vi "Read Encoders.vi"(8 "Reset":bool, 10 "Right Encoder":T2, 11 "Left Encoder":T2) -> (0 "Encoder Values":T1, 2 "Right Encoder Out":T2, 3 "Left Encoder Out":T2)   [LabVIEW 2013]
uses:
  <vilib>/Rock Robotics/WPI/Encoder/WPI_EncoderDevRef.ctl
  <vilib>/Rock Robotics/SystemInterfaces/Encoder/FPGA_EncoderIdx.ctl
  <vilib>/Rock Robotics/SystemInterfaces/Counter/FPGA_CounterCtrSystemIndex.ctl
  <vilib>/Rock Robotics/WPI/Encoder/WPI_EncoderType.ctl
  Encoder Values.ctl
  <vilib>/addons/control/pid/pid.llb/PID Control Input Filter (DBL).vi
  <vilib>/addons/control/pid/NI_PID_pid.lvlib
panel:
  in  "Left constant":dbl=0.00724
  in  "Right constant":dbl=0.00724
  in  "Right tick constant":dbl=0.697
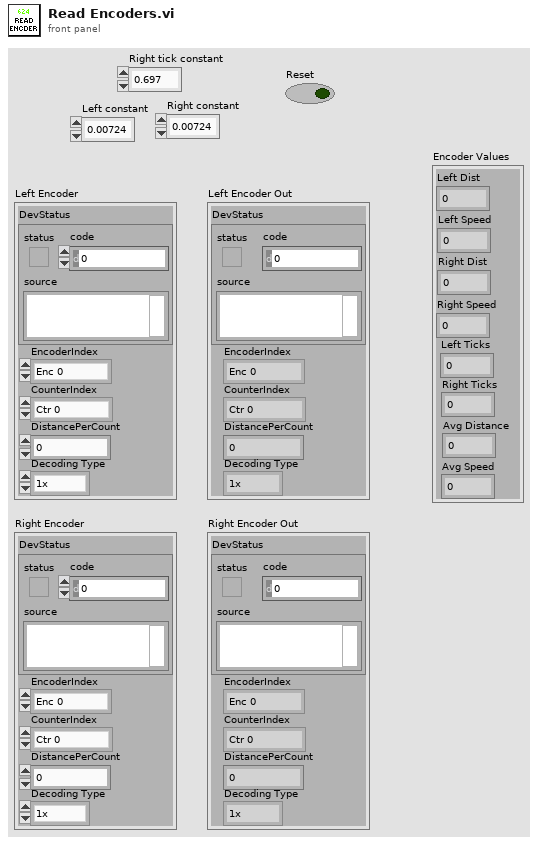
[diagram p1: front panel]
types:
  T1 = typedef "Encoder Values.ctl" = cluster{"Left Dist":dbl, "Left Speed":dbl, "Right Dist":dbl, "Right Speed":dbl, "Left Ticks":dbl, "Right Ticks":dbl, "Avg Distance":dbl, "Avg Speed":dbl}
  T2 = typedef "WPI_EncoderDevRef.ctl" = cluster{"DevStatus":errorcluster, "EncoderIndex":T3, "CounterIndex":T4, "DistancePerCount":dbl, "Decoding Type":T5}
  T3 = typedef "FPGA_EncoderIdx.ctl" = enum8{"Enc 0", "Enc 1", "Enc 2", "Enc 3", "Invalid"}
  T4 = typedef "FPGA_CounterCtrSystemIndex.ctl" = enum8{"Ctr 0", "Ctr 1", "Ctr 2", "Ctr 3", "Ctr 4", "Ctr 5", "Ctr 6", "Ctr 7", "Invalid"}
  T5 = typedef "WPI_EncoderType.ctl" = enum16{"1x", "2x", "4x"}
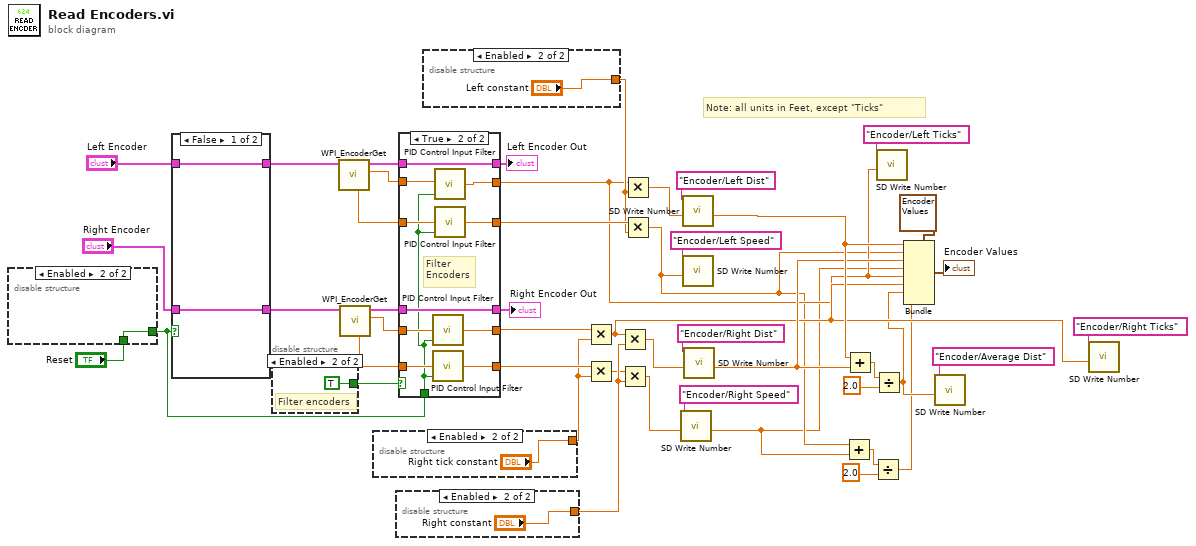
[diagram p0: block diagram]
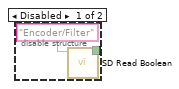
[diagram p2: hidden frame]
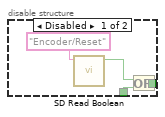
[diagram p3: hidden frame]
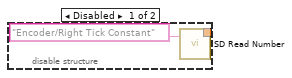
[diagram p4: hidden frame]
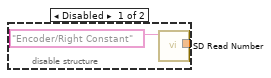
[diagram p5: hidden frame]
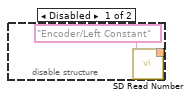
[diagram p6: hidden frame]
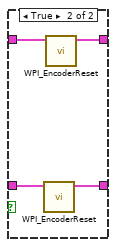
[diagram p7: hidden frame]
diagram:
  # "Note: all units in Feet, except \"Ticks\""
  n1 = disable-structure shown="Enabled" {
    disable-tunnel: "Reset" -> [w46 w48]
    disable-tunnel: [w44 w48] -> w7
    frame Disabled {
      n2 = call <vilib>:"SD Read Boolean.vi"("Name"="Encoder/Reset") -> ("Boolean"=w45:bool)  [unwired: 8 in, 2 out]
      n3 = Or(x=w45, y=w46) -> (x .or. y?=w44:bool)
    }
    frame Enabled {
    }
  }
  n4 = case shown="False" w7 {
    tunnel: [w49 w54] -> w8
    tunnel: [w50 w53] -> w9
    tunnel: "Left Encoder" -> [w50 w52]
    tunnel: "Right Encoder" -> [w49 w51]
    frame False {
    }
    frame True {
      n5 = call <vilib>:"WPI_EncoderReset.vi"("EncoderDevRef"=w51) -> ("EncoderDevRef"=w54:T2)  [unwired: 9 in, 1 out]
      n6 = call <vilib>:"WPI_EncoderReset.vi"("EncoderDevRef"=w52) -> ("EncoderDevRef"=w53:T2)  [unwired: 9 in, 1 out]
    }
  }
  n7 = disable-structure shown="Enabled" {
    disable-tunnel: [w55 TRUE ("Boolean")] -> w12
    frame Disabled {
      n8 = call <vilib>:"SD Read Boolean.vi"("Name"="Encoder/Filter") -> ("Boolean"=w55:bool)  [unwired: 8 in, 2 out]
    }
    frame Enabled {
      # "Filter encoders"
    }
  }
  n9 = call <vilib>:"WPI_EncoderGet.vi"("EncoderDevRef"=w9) -> ("Distance"=w33:dbl, "EncoderDevRef"=w36:T2, "Rate"=w34:dbl)  [unwired: 5 in, 3 out]
  n10 = call <vilib>:"WPI_EncoderGet.vi"("EncoderDevRef"=w8) -> ("Distance"=w32:dbl, "EncoderDevRef"=w35:T2, "Rate"=w31:dbl)  [unwired: 5 in, 3 out]
  n11 = disable-structure shown="Enabled" {
    disable-tunnel: [w58 "Right tick constant"] -> w24
    frame Disabled {
      n12 = call <vilib>:"SD Read Number.vi"("Name"="Encoder/Right Tick Constant") -> ("Numeric"=w58:dbl)  [unwired: 8 in, 2 out]
    }
    frame Enabled {
    }
  }
  n13 = disable-structure shown="Enabled" {
    disable-tunnel: [w61 "Right constant"] -> w27
    frame Disabled {
      n14 = call <vilib>:"SD Read Number.vi"("Name"="Encoder/Right Constant") -> ("Numeric"=w61:dbl)  [unwired: 8 in, 2 out]
    }
    frame Enabled {
    }
  }
  n15 = case shown="True" w12 {
    tunnel: w36 -> [w69 w80]
    tunnel: w35 -> [w66 w79]
    tunnel: [w69 w80] -> w15
    tunnel: [w66 w79] -> w16
    tunnel: w33 -> [w68 w78]
    tunnel: w34 -> [w67 w77]
    tunnel: [w67 w76] -> w30
    tunnel: [w68 w75] -> w19
    tunnel: w31 -> [w64 w74]
    tunnel: w32 -> [w65 w73]
    tunnel: [w65 w72] -> w23
    tunnel: [w64 w71] -> w26
    tunnel: w7 -> [_ w70]
    frame False {
      # "No filtering"
    }
    frame True {
      # "Filter\nEncoders"
      n16 = call-poly <vilib>:"PID Control Input Filter.vi"("reinitialize? (F)"=w70, "input"=w73) -> ("output"=w72:dbl)  [unwired: 3 in]
      n17 = call-poly <vilib>:"PID Control Input Filter.vi"("reinitialize? (F)"=w70, "input"=w74) -> ("output"=w71:dbl)  [unwired: 3 in]
      n18 = call-poly <vilib>:"PID Control Input Filter.vi"("reinitialize? (F)"=w70, "input"=w78) -> ("output"=w75:dbl)  [unwired: 3 in]
      n19 = call-poly <vilib>:"PID Control Input Filter.vi"("reinitialize? (F)"=w70, "input"=w77) -> ("output"=w76:dbl)  [unwired: 3 in]
    }
  }
  "Right Encoder Out" <- w16
  "Left Encoder Out" <- w15
  n20 = disable-structure shown="Enabled" {
    disable-tunnel: [w82 "Left constant"] -> w28
    frame Disabled {
      n21 = call <vilib>:"SD Read Number.vi"("Name"="Encoder/Left Constant") -> ("Numeric"=w82:dbl)  [unwired: 8 in, 2 out]
    }
    frame Enabled {
    }
  }
  n22 = Multiply(x=w23, y=w24) -> (x*y=w20:dbl)
  n23 = Multiply(x=w26, y=w24) -> (x*y=w25:dbl)
  n24 = Multiply(x=w20, y=w27) -> (x*y=w21:dbl)
  n25 = Multiply(x=w25, y=w27) -> (x*y=w2:dbl)
  n26 = Multiply(x=w19, y=w28) -> (x*y=w29:dbl)
  n27 = Multiply(x=w30, y=w28) -> (x*y=w3:dbl)
  n28 = call <vilib>:"SD Write Number.vi"("Numeric"=w2, "Name"="Encoder/Right Speed") -> ()  [unwired: 8 in, 2 out]
  n29 = call <vilib>:"SD Write Number.vi"("Numeric"=w29, "Name"="Encoder/Left Dist") -> ()  [unwired: 8 in, 2 out]
  n30 = call <vilib>:"SD Write Number.vi"("Numeric"=w3, "Name"="Encoder/Left Speed") -> ()  [unwired: 8 in, 2 out]
  n31 = call <vilib>:"SD Write Number.vi"("Numeric"=w21, "Name"="Encoder/Right Dist") -> ()  [unwired: 8 in, 2 out]
  n32 = Add(x=w3, y=w2) -> (x+y=w5:dbl)
  n33 = Add(x=w29, y=w21) -> (x+y=w38:dbl)
  n34 = Divide(x=w5, y=2.0) -> (x/y=w1:dbl)
  n35 = Divide(x=w38, y=2.0) -> (x/y=w17:dbl)
  n36 = call <vilib>:"SD Write Number.vi"("Numeric"=w19, "Name"="Encoder/Left Ticks") -> ()  [unwired: 8 in, 2 out]
  n37 = Bundle(cluster=T1 {"Left Dist"=-0.6624599999999999, "Left Speed"=0.0, "Right Dist"=-0.6850325099999999, "Right Speed"=0.0, "Left Ticks"=-91.5, "Right Ticks"=-94.61774999999999, "Avg Distance"=-94.61774999999999, "Avg Speed"=0.0} ("output cluster"), "Left Dist"=w29, "Left Speed"=w3, "Right Dist"=w21, "Right Speed"=w2, "Left Ticks"=w19, "Right Ticks"=w20, "Avg Distance"=w17, "Avg Speed"=w1) -> (→"Encoder Values":T1)
  n38 = call <vilib>:"SD Write Number.vi"("Numeric"=w17, "Name"="Encoder/Average Dist") -> ()  [unwired: 8 in, 2 out]
  n39 = call <vilib>:"SD Write Number.vi"("Numeric"=w20, "Name"="Encoder/Right Ticks") -> ()  [unwired: 8 in, 2 out]
